vi "Clear Selection.vi"(8 "error in (no error)":errorcluster, 11 "Editor in":refnum<class "Editor.lvclass">) -> (0 "error out":errorcluster, 3 "Editor out":refnum<class "Editor.lvclass">)   [LabVIEW 2020, in "VolatusGUIEditor.lvlib" / "Editor.lvclass"]
uses:
  Editor.lvclass
  Editor.lvclass/Editor.ctl
  lv-oopanel/OOPanel/Manager/Manager.lvclass
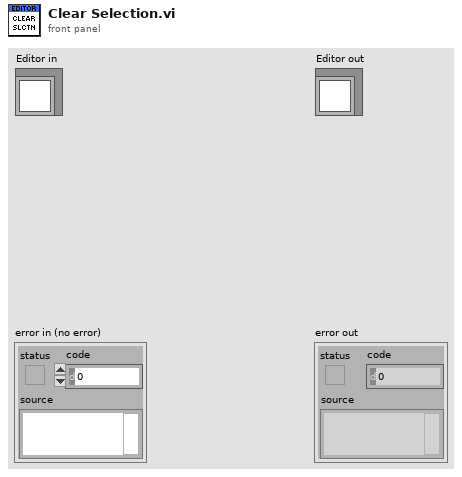
[diagram p1: front panel]
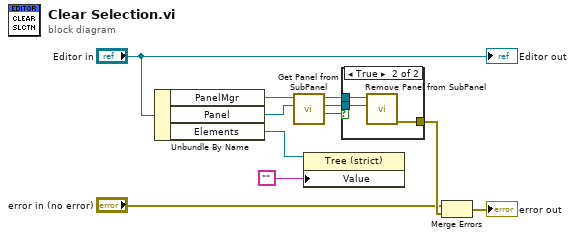
[diagram p0: block diagram]
diagram:
  n1 = Unbundle By Name("Editor in") -> ("PanelMgr"=w10:refnum<class "Manager.lvclass">, "Panel"=w9:refnum<vi>, "Elements"=w2:refnum<vi>)
  n2 = call "Get Panel from SubPanel.vi"("SubPanel"=w9, "Manager in"=w10) -> ("Has Panel"=w6:bool, "Panel"=w7:refnum<class "Panel.lvclass">, "Manager out"=w8:refnum<class "Manager.lvclass">)  [unwired: 6 in, 1 out]
  n3 = property class="Tree (strict)"(reference=w2, "Value"="") -> ()  [unwired: 1 in, 2 out]
  n4 = case shown="True" w6 {
    tunnel: w8 -> [_ w14]
    tunnel: w7 -> [_ w13]
    tunnel: [_ w12] -> w4
    frame False {
    }
    frame True {
      n5 = call "Remove Panel from SubPanel.vi"("Panel In"=w13, "Manager in"=w14) -> ("error out"=w12:errorcluster)  [unwired: 7 in, 2 out]
    }
  }
  n6 = Merge Errors("error in (no error)", w4) -> (→"error out":errorcluster)
  "Editor out" <- "Editor in"
